vi "make_metadata_array.vi"(3 "Cluster":T1 {"File Location" items=["Unknown"=-1, "Storage"=0, "Processing"=1]; "Estimate Source" items=["Any Source."=-2, "No Shot"=-1, "Basic Labview Estimate"=0, "IDL Estimate From Andrew"=1, "IDL Estimate From Tobin"=2, "Old Metadata"=3]}) -> (0 "Metadata Array":string[](array[string]), 1 "Header Array":string[](array[string]))   [LabVIEW 2013]
uses:
  User Interface/Controls/Query_Dust_Event.ctl
  User Interface/Controls/Estimate_source.ctl
  User Interface/Controls/File_location.ctl
panel:
  # "Dust Event"
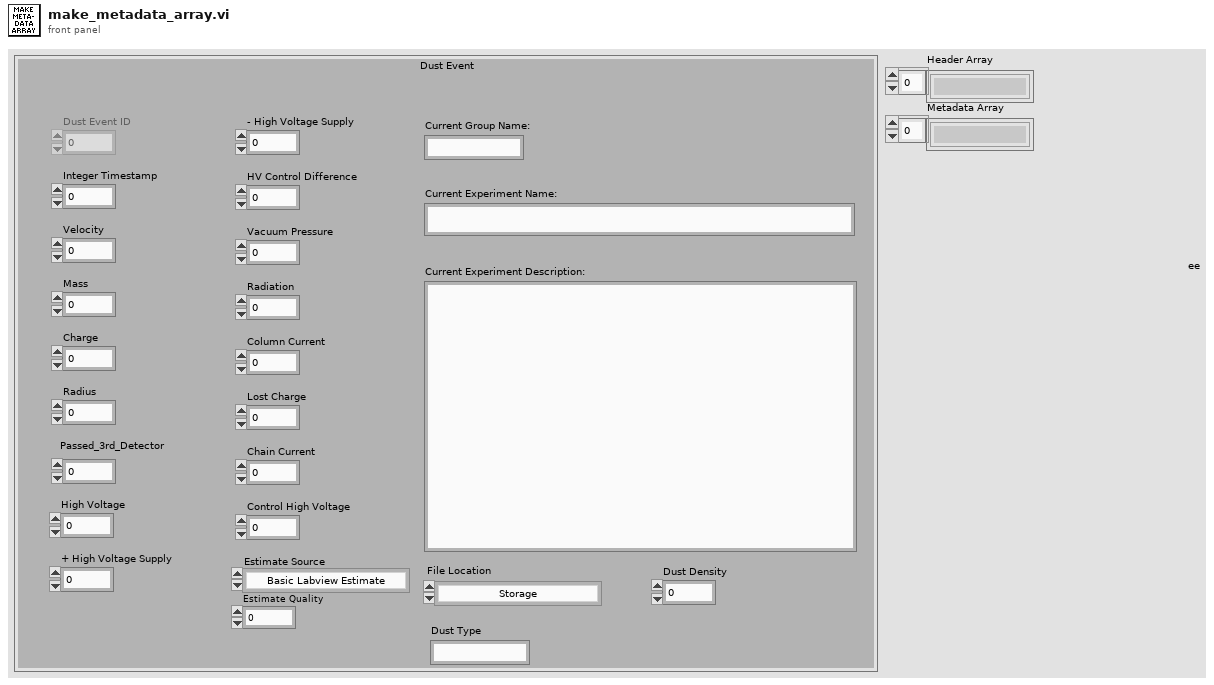
[diagram p1: front panel]
types:
  T1 = typedef "Query_Dust_Event.ctl" = cluster{"Dust Event ID":i64, "Integer Timestamp":i64, "Velocity":dbl, "Mass":dbl, "Charge":sgl, "Radius":sgl, "Passed_3rd_Detector":i8, "High Voltage":sgl, "+ High Voltage Supply":sgl, "- High Voltage Supply":sgl, "HV Control Difference":sgl, "Vacuum Pressure":sgl, "Radiation":sgl, "Column Current":sgl, "Lost Charge":sgl, "Chain Current":sgl, "Control High Voltage":sgl, "Current Group Name:":string, "Current Experiment Name:":string, "Current Experiment Description:":string, "Estimate Source":T2, "Estimate Quality":i8, "File Location":T3, "Dust Type":string, "Dust Density":sgl}
  T2 = typedef "Estimate_source.ctl" = i8
  T3 = typedef "File_location.ctl" = i8
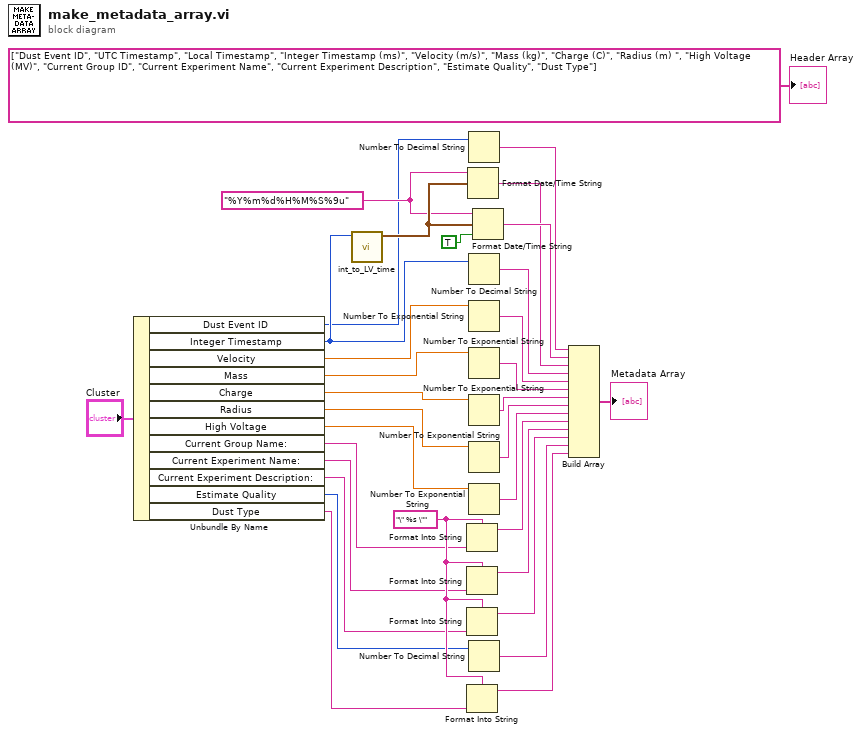
[diagram p0: block diagram]
diagram:
  w28 = "\" %s \"" ("format string")
  w30 = "%Y%m%d%H%M%S%9u" ("time format string (%c)")
  n1 = Unbundle By Name("Cluster") -> ("Dust Event ID"=w11:i64, "Integer Timestamp"=w18:i64, "Velocity"=w12:dbl, "Mass"=w13:dbl, "Charge"=w17:sgl, "Radius"=w14:sgl, "High Voltage"=w15:sgl, "Current Group Name:"=w24:string, "Current Experiment Name:"=w22:string, "Current Experiment Description:"=w20:string, "Estimate Quality"=w16:i8, "Dust Type"=w26:string)
  n2 = call "int_to_LV_time.vi"("Integer Timestamp"=w18) -> ("time stamp"=w31:timestamp)  [unwired: 8 in, 1 out]
  n3 = Format Into String(format string=w28, w24) -> (resulting string=w25:string)  [unwired: 2 in, 1 out]
  n4 = Format Into String(format string=w28, w22) -> (resulting string=w23:string)  [unwired: 2 in, 1 out]
  n5 = Format Into String(format string=w28, w20) -> (resulting string=w21:string)  [unwired: 2 in, 1 out]
  n6 = Format Into String(format string=w28, w26) -> (resulting string=w27:string)  [unwired: 2 in, 1 out]
  n7 = Format Date/Time String(time format string (%c)=w30, seconds (now)=w31) -> (date/time string=w19:string)  [unwired: 1 in]
  n8 = Number To Decimal String(number=w11) -> (decimal integer string=w29:string)  [unwired: 1 in]
  n9 = Number To Decimal String(number=w18) -> (decimal integer string=w4:string)  [unwired: 1 in]
  n10 = Number To Exponential String(number=w12) -> (E-format string=w5:string)  [unwired: 3 in]
  n11 = Number To Exponential String(number=w13) -> (E-format string=w6:string)  [unwired: 3 in]
  n12 = Number To Exponential String(number=w17) -> (E-format string=w7:string)  [unwired: 3 in]
  n13 = Number To Exponential String(number=w14) -> (E-format string=w8:string)  [unwired: 3 in]
  n14 = Number To Exponential String(number=w15) -> (E-format string=w9:string)  [unwired: 3 in]
  n15 = Number To Decimal String(number=w16) -> (decimal integer string=w10:string)  [unwired: 1 in]
  n16 = Format Date/Time String(time format string (%c)=w30, seconds (now)=w31, UTC format=TRUE) -> (date/time string=w33:string)
  n17 = Build Array(w29, w33, w19, w4, w5, w6, w7, w8, w9, w25, w23, w21, w10, w27) -> (→"Metadata Array":string[])
  "Header Array" <- string[] ["Dust Event ID", "UTC Timestamp", "Local Timestamp", "Integer Timestamp (ms)", "Velocity (m/s)", "Mass (kg)", "Charge (C)", "Radius (m) ", "High Voltage (MV)", "Current Group ID", "Current Experiment Name", "Current Experiment Description", "Estimate Quality", "Dust Type"]
